vi "Create Pattern Script - Rd Compare Frame.vi"(8 "error in (no error)":errorcluster, 10 "FRM Data":T1 {"Addr" format="%x"; "Data" format="%x"}, 11 "SPI 4W Pattern Creator in":refnum<class "SPI 4W Pattern Creator.lvclass">) -> (0 "error out":errorcluster, 2 "String":string, 3 "SPI 4W Pattern Creator out":refnum<class "SPI 4W Pattern Creator.lvclass">)   [LabVIEW 2018, in "SPI 4W Pattern Creator.lvlib" / "SPI 4W Pattern Creator.lvclass"]
uses:
  SPI 4W Pattern Creator.lvclass
  Ctls/Frame Data - SPI_3W.ctl
  Ctls/RW Options.ctl
  Protocols/SPI Root Pattern Creator.lvlibp/Plugins/SouceCode/SPI_Pattern Creator/SPI Root/Data Type.ctl
  Protocols/SPI Root Pattern Creator.lvlibp/Plugins/SouceCode/SPI_Pattern Creator/SPI Root/Special Frame Type.ctl
  Protocols/SPI Root Pattern Creator.lvlibp/Plugins/SouceCode/SPI_Pattern Creator/SPI Root/SPI Root Pattern Creator.lvclass
  C:/P4 Workspace/PC Client/Solutions/5g_eap/trunk/1.0/HiSi5GmmWave/Pattern_Gen_Tool/Plugins/Protocols/SPI Root Pattern Creator.lvlibp/Plugins/SouceCode/SPI_Pattern Creator/SPI Root/SPI Root Pattern Creator.lvclass
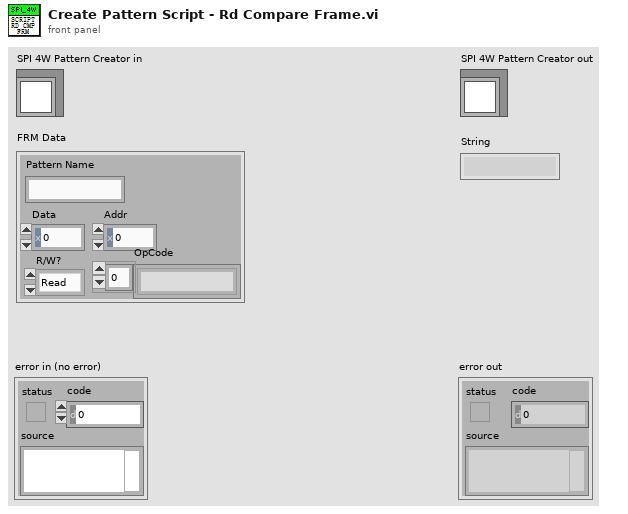
[diagram p1: front panel]
types:
  T1 = typedef "Frame Data - SPI_3W.ctl" = cluster{"Pattern Name":string, "Data":u16, "Addr":u16, "OpCode":string[], "R/W?":T2}
  T2 = typedef "RW Options.ctl" = enum16{"Read", "Write", "R/W"}
  T3 = typedef "SPI Root Pattern Creator.lvlibp/SPI Root Pattern Creator.lvclass/Special Frame Type.ctl" = enum16{"SPI 4W FRM Start", "SPI 4W Wait", "SPI 4W FRM End", "SPI 4W Write Cmd", "SPI Rd Collect Cmd", "SPI Rd Value Cmd", "SPI 3W FRM Start", "SPI 3W Write Cmd", "SPI 3W FRM End", "SPI 3W Wait", "SPI 3W Rd Cmd"}
  T4 = typedef "SPI Root Pattern Creator.lvlibp/SPI Root Pattern Creator.lvclass/Data Type.ctl" = enum16{"Drive", "Compare", "Read"}
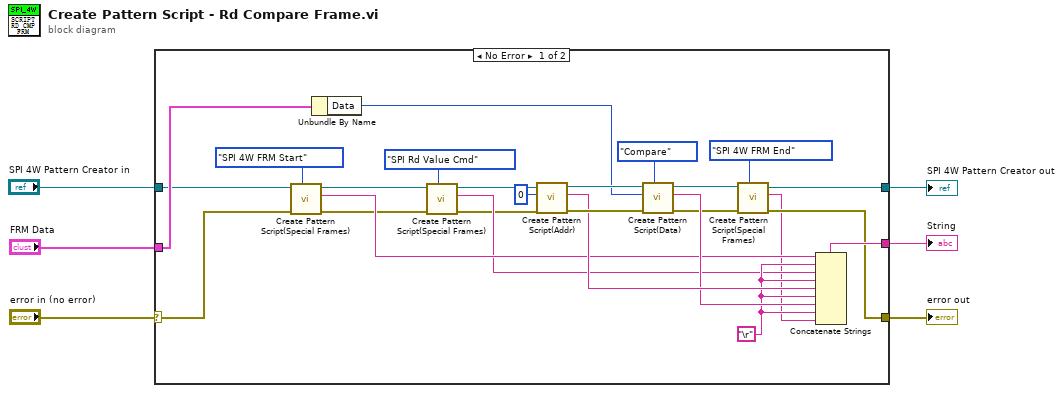
[diagram p0: block diagram]
diagram:
  n1 = case shown="No Error" "error in (no error)" {
    selector: "error in (no error)" -> [w23 w33]
    tunnel: "FRM Data" -> [w32 _]
    tunnel: "SPI 4W Pattern Creator in" -> [w22 w34]
    tunnel: [w11 w34] -> w3
    tunnel: [w13 w33] -> w1
    tunnel: [w26 _] -> w2
    frame No Error {
      w27 = "\r"
      n2 = call "Create Pattern Script(Special Frames).vi"("Special Frame Type"=Special_Frame_Type."SPI 4W FRM Start", "error in (no error)"=w23, "SPI Root Pattern Creator in"=w22) -> ("error out"=w19:errorcluster, "String out"=w21:string, "SPI Root Pattern Creator out"=w20:refnum<class "SPI 4W Pattern Creator.lvclass">)  [unwired: 6 in]
      n3 = Unbundle By Name(w32) -> ("Data"=w24:u16)
      n4 = call "Create Pattern Script(Special Frames).vi"("Special Frame Type"=Special_Frame_Type."SPI Rd Value Cmd", "error in (no error)"=w19, "SPI Root Pattern Creator in"=w20) -> ("error out"=w16:errorcluster, "String out"=w17:string, "SPI Root Pattern Creator out"=w18:refnum<class "SPI 4W Pattern Creator.lvclass">)  [unwired: 6 in]
      n5 = call-dynamic "Create Pattern Script(Addr).vi"("error in (no error)"=w16, "Addr"=u16 0, "SPI 4W Pattern Creator in"=w18) -> ("error out"=w31:errorcluster, "String"=w29:string, "SPI 4W Pattern Creator out"=w30:refnum<class "SPI 4W Pattern Creator.lvclass">)  [unwired: 6 in]
      n6 = call-dynamic "Create Pattern Script(Data).vi"("Data Type"=Data_Type."Compare", "error in (no error)"=w31, "Data"=w24, "SPI 4W Pattern Creator in"=w30) -> ("error out"=w14:errorcluster, "String"=w28:string, "SPI 4W Pattern Creator out"=w15:refnum<class "SPI 4W Pattern Creator.lvclass">)  [unwired: 5 in]
      n7 = call "Create Pattern Script(Special Frames).vi"("Special Frame Type"=Special_Frame_Type."SPI 4W FRM End", "error in (no error)"=w14, "SPI Root Pattern Creator in"=w15) -> ("error out"=w13:errorcluster, "String out"=w12:string, "SPI Root Pattern Creator out"=w11:refnum<class "SPI 4W Pattern Creator.lvclass">)  [unwired: 6 in]
      n8 = Concatenate Strings(w21, w27, w17, w27, w29, w27, w28, w27, w12) -> (w26:string)
    }
    frame Error {
    }
  }
  "error out" <- w1
  "SPI 4W Pattern Creator out" <- w3
  "String" <- w2
